vi "NI 5772 (AC) - Digitizer_(FPGA)Averaging (Working).vi"() -> ()   [LabVIEW 2020]
doc: "Example Description:\nThis example demonstrates how to enable Time Interleaved Sampling with the NI 5772 adapter module to achieve a sampling rate of 1.6GS/s. This example continuously acquires records of analog input data from the NI 5772 adapter module. It allows you to select an AI channel, trigger type, and record size. This VI must be compiled before it is run. \n\nRunning the VI:\nThis VI must be run from the NI 5772 - Getting Started (Host).vi. Refer to the host VI documentation for steps regarding running and configuring the FPGA VI. \n\nExecution Steps:\nRefer to the Block Diagram of this VI for execution comments."
uses:
  Controls/AI Trigger Type.ctl
  Controls/Aquire State.ctl
  <vilib>/Platform/TimedLoop/XDataNode/timing_clust.ctl
  <vilib>/Platform/TimedLoop/XDataNode/nitl_modes.ctl
  <vilib>/Platform/TimedLoop/XDataNode/wakeup.ctl
  Controls/DigitizerState.ctl
  <vilib>/rvi/Emulation/niFpgaGetClockAttributes.vi
  <vilib>/rvi/Emulation/niFpgaSctlEmulationGetInTimedLoop.vi
  <vilib>/rvi/Emulation/niFpgaEmulationReportErrorSimple.vi
  <vilib>/rvi/eio/common/nirviEmuTemplateMethod_errors.vi
  <vilib>/rvi/Emulation/niFpgaCriticalErrorInLSC.vi
  <vilib>/rvi/Emulation/niFpgaProcessEmulError.vi
  <vilib>/rvi/Emulation/niFpgaEmulationIsFPGAContextNoSignature.vi
  <vilib>/rvi/errors/niFpgaSetErrorForExecOnDevCompSimple.vi
  <vilib>/rvi/eio/common/nirviEmuReportErrorAndStop.vi
  <vilib>/rvi/DataTransferAndStorage/Container/Common/niFpgaContainerGetUniqueNameForEmu.vi
  <vilib>/rvi/FIFO/Fifo_Resource/nirvififoEmulationSetSize.vi
  <vilib>/rvi/FIFO/Fifo_Resource/nirviFifoEmulationQueueMgr.vi
  <instcachedir>/0/nirviFifoEmulationQueueMgr_E5CAEC123FF24DC58D834DCA3CDAA9B5.lvgen/nirviFifoEmulationQueueMgr_E5CAEC123FF24DC58D834DCA3CDAA9B5_000.vi
  <vilib>/Utility/error.llb/Clear Errors.vi
  <vilib>/rvi/FIFO/Fifo_Resource/nirvififoEmulationCreateLock.vi
  <vilib>/rvi/FIFO/Fifo_Resource/nirvififoEmulationObtainLock.vi
  <vilib>/rvi/FIFO/Fifo_Resource/nirvififoEmulationReleaseLock.vi
  <vilib>/rvi/occurrence/nirviWaitOnOccurrenceBase.vi
  <vilib>/rvi/errors/nirviReportUnexpectedCaseInternalError.vi
  <vilib>/rvi/errors/nirviReportUnexpectedCaseInternalError (U32).vi
  <instcachedir>/0/nirviFifoEmulationQueueMgr_E5CAEC123FF24DC58D834DCA3CDAA9B5.lvgen/nirviFifoEmulationQueueMgr_E5CAEC123FF24DC58D834DCA3CDAA9B5_003.vi
  <vilib>/rvi/FIFO/Fifo_Resource/nirvififoEmulationDetermineInputValidOut.vi
  <vilib>/rvi/Memory/Memory_Emulation/nirvimemoryFastEmulation.vi
  <vilib>/rvi/Memory/Memory_Emulation/nirvimemoryEmulation.vi
  <vilib>/rvi/interface/RandomDataEmulation/niFpgaRandomDataHandleErrors.vi
  <instcachedir>/0/nirviFifoEmulationQueueMgr_E5CAEC123FF24DC58D834DCA3CDAA9B5.lvgen/nirviFifoEmulationQueueMgr_E5CAEC123FF24DC58D834DCA3CDAA9B5_004.vi
  <instrlib>/_niInstr/Basic Elements/v1/FPGA/Private/Count Up U64.vi
  <vilib>/eio/EIONode/EIONode.xnode
  <vilib>/Platform/TimedLoop/XDataNode/XDataNode.xnode
  <vilib>/rvi/DataTransferAndStorage/Container/XNode/niFpgaContainer.xnode
  <vilib>/rvi/FIFO/Fifo_Resource/nirvififoEmulationRead.vi
  <vilib>/rvi/FIFO/Fifo_Resource/nirvififoEmulationWrite.vi
  <vilib>/rvi/interface/RandomDataEmulation/nirviRandomDataFpgaReadWriteTemplate.vi
  <vilib>/Platform/TimedLoop/XDataNode/XDNodeRunTimeDep.lvlib
  <instrlib>/_niInstr/Basic Elements/v1/FPGA/niInstr Basic Elements v1 FPGA.lvlib
panel:
  in  "Pulse Width Off [cycles]":u16=5
  in  "Pulse Width On [cycles]":u16=10
  out "Read Size (Host)":u16=512 caption="Samples Per Trigger" min=1 step=1
  out "Trig Count":u64
  in  "Clear Count":bool
  in  "TrigIn Simulate":bool
  in  "vi/nGenTrig":bool
  in  "Arm Trigger":bool
  out "F to H FIFO Overflow?":bool caption="FIFO Overflow?"
  out "DataAlignmentFIFO":bool
  out "Aq to Trans FIFO Overflow?":bool caption="FIFO Overflow?"
  in  "Requested Samples Per Pixel":u16=512 caption="Samples Per Trigger" min=1 step=1
  in  "AvgCount_powerOf2":i16=1
  in  "Delay (us)":sgl
  in  "WaveSampleCount":sgl=256.0 format="%#_13g"
  in  "Wave Sampling Rate":sgl=200000000.0 format="%#_6p"
  in  "Trigger Level":i16
  in  "Trigger Type":T1
  out "AvgCount":u16=1
  out "Delay after Trig [cycles]":u16
  out "1/8th Samples Per Trigger":u16=512 caption="Samples Per Trigger" min=1 step=1
  out "WaitForWave\nCompletion [cycles]":u16
  in  "User Command Commit":bool
  in  "User Command":u8
  out "User Command Idle":bool
  out "User Command Status":u8
  in  "User Data 0":u16
  in  "User Data 1":u8
  out "PLL Locked":bool
  out "User Error":bool
  out "Configured?":bool
  # "Trigger Settings"
  # "FIFO Status"
  # "Analog Input"
  # "Clock Configuration"
  # "Resource Configuration"
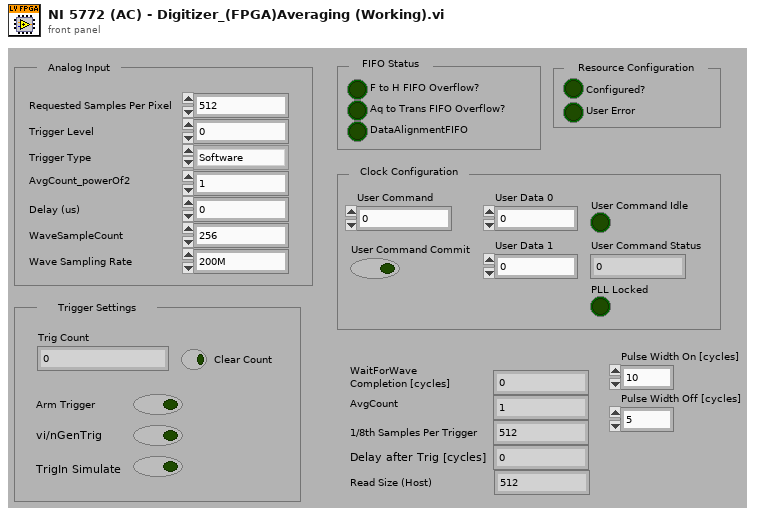
[diagram p1: front panel]
types:
  T1 = typedef "AI Trigger Type.ctl" = enum8{"Software", "Data Edge"}
  T2 = typedef "DigitizerState.ctl" = enum16{"Init", "Build/Clear Accumulator", "GetData", "SetData", "AverageCountCheck", "SendtoHost"}
  T3 = typedef "Aquire State.ctl" = enum8{"Idle", "Wait for Trigger", "AlignWave", "Hold Aquire", "Acquire", "WaitForWaveCompletion", "CheckAvg"}
  T4 = typedef "XDNodeRunTimeDep.lvlib/timing_clust.ctl" = cluster{"Expected End [f-1]":u64, "Actual End [f-1]":u64, "Finished Late? [f-1]":bool, "Expected End [i-1]":u64, "Actual End [i-1]":u64, "Finished Late? [i-1]":bool, "Expected Start [i]":u64, "Actual Start [i]":u64, "Expected Start [f]":u64, "Actual Start [f]":u64, "Source Name":string, "Structure Name":string, "Period":i64, "Deadline":i64, "Offset":i64, "Start":i64, "Priority":i32, "Timeout":i32, "Mode":T5, "Wakeup Reason":T6, "Error":errorcluster, "Source Type":string, "Secondary Source Type":string, "Global End Time":u64, "Global Start Time":u64, "Frame Duration":u64, "Iteration Duration":u64, "Assigned CPU":i32, "I/O Scan Engine Mode":u32}
  T5 = typedef "XDNodeRunTimeDep.lvlib/nitl_modes.ctl" = enum32{"No Change", "Process missed periods, maintain original phase", "Discard missed periods, maintain original phase", "Process missed periods, ignore original phase", "Discard missed periods, ignore original phase"}
  T6 = typedef "XDNodeRunTimeDep.lvlib/wakeup.ctl" = enum32{"Normal", "Aborted", "Asynchronous wakeup", "Timing source error", "Timed loop error", "Timeout"}
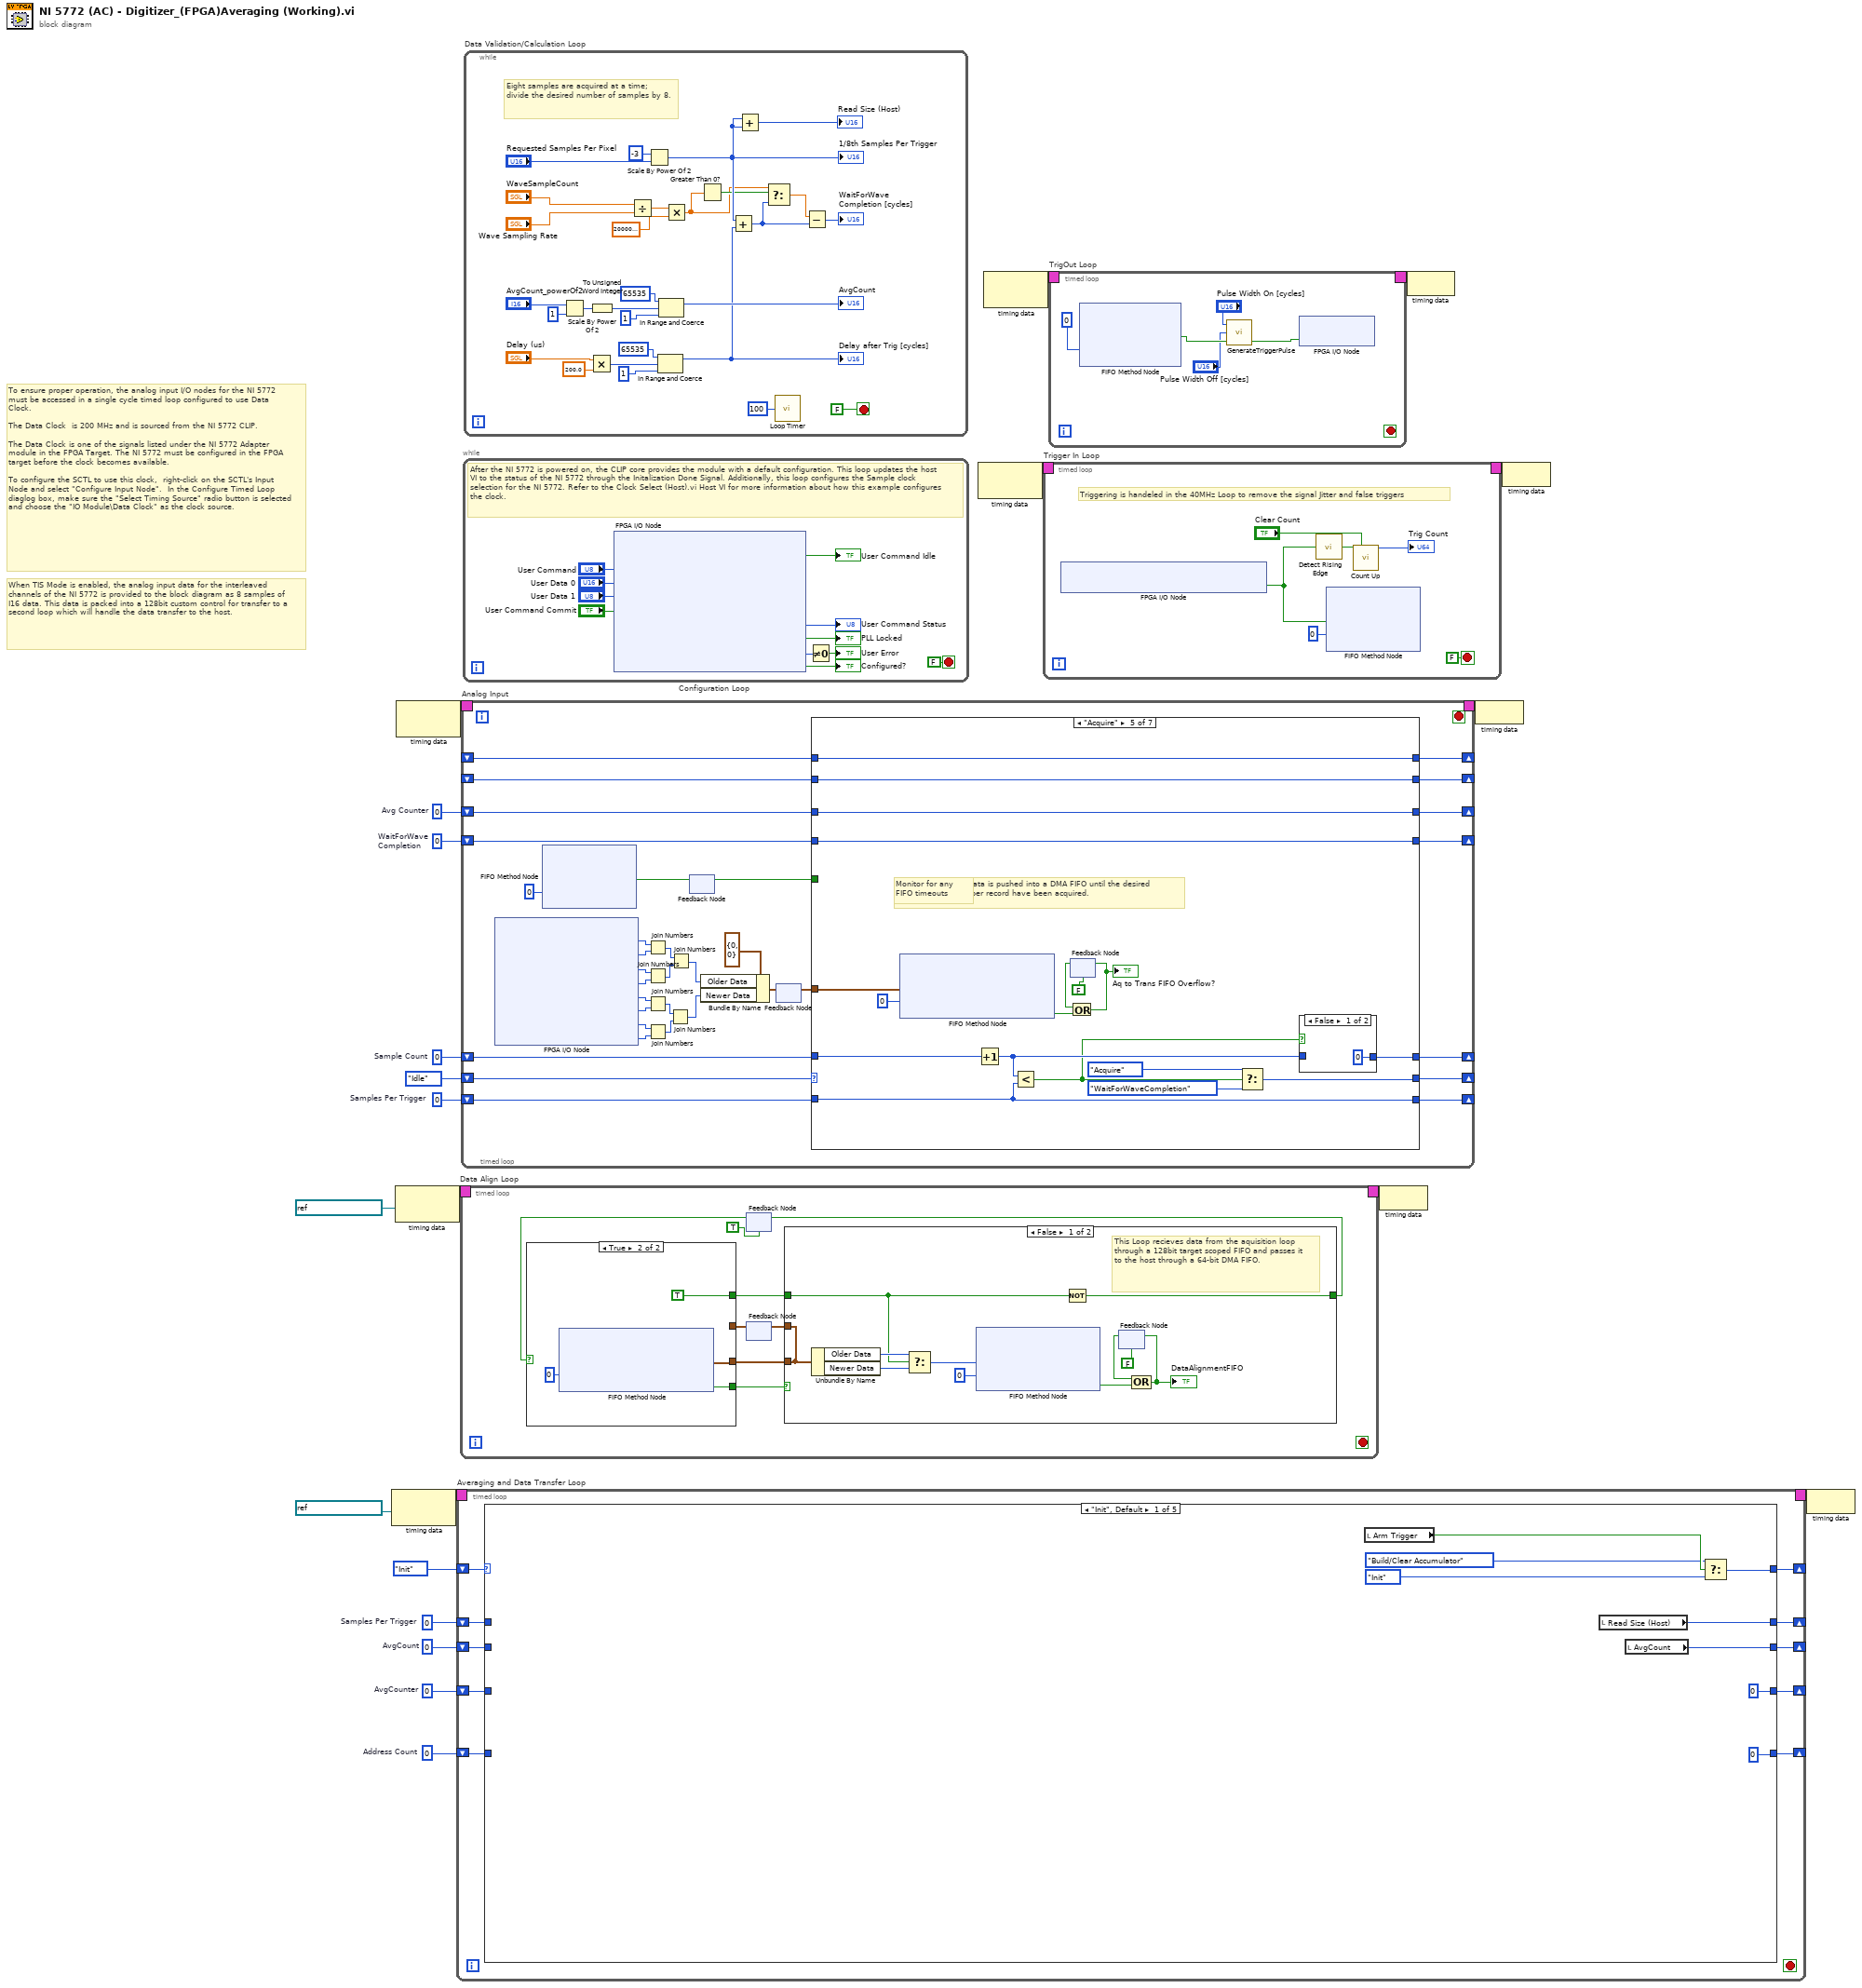
[diagram p0: block diagram]
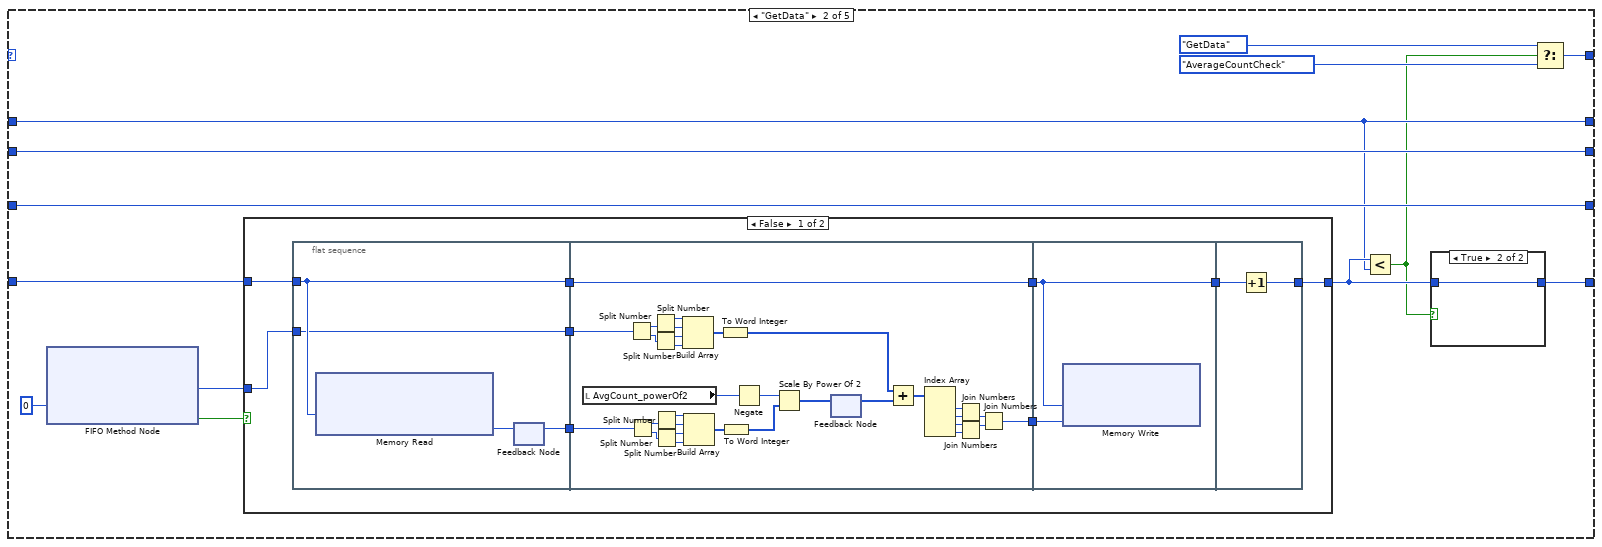
[diagram p2: hidden frame]
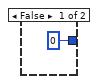
[diagram p3: hidden frame]
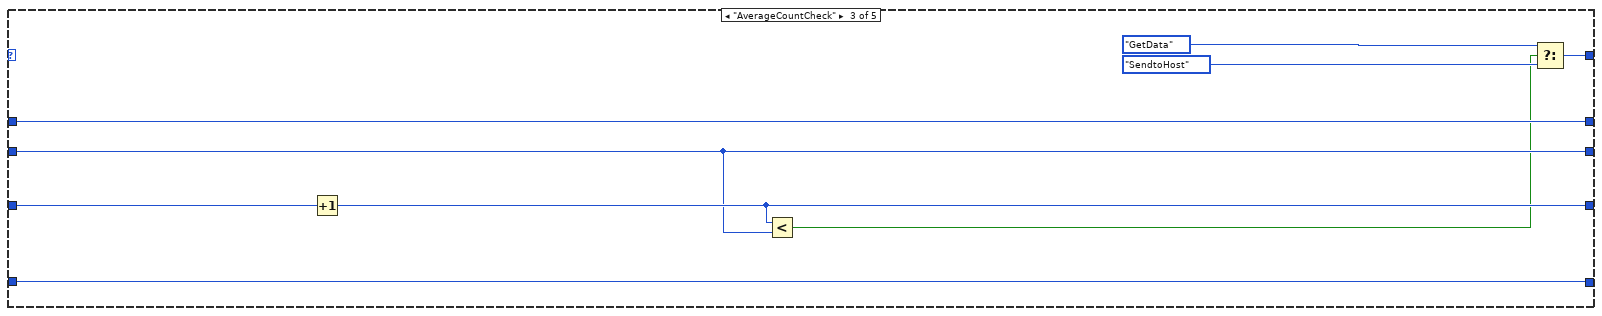
[diagram p5: hidden frame]
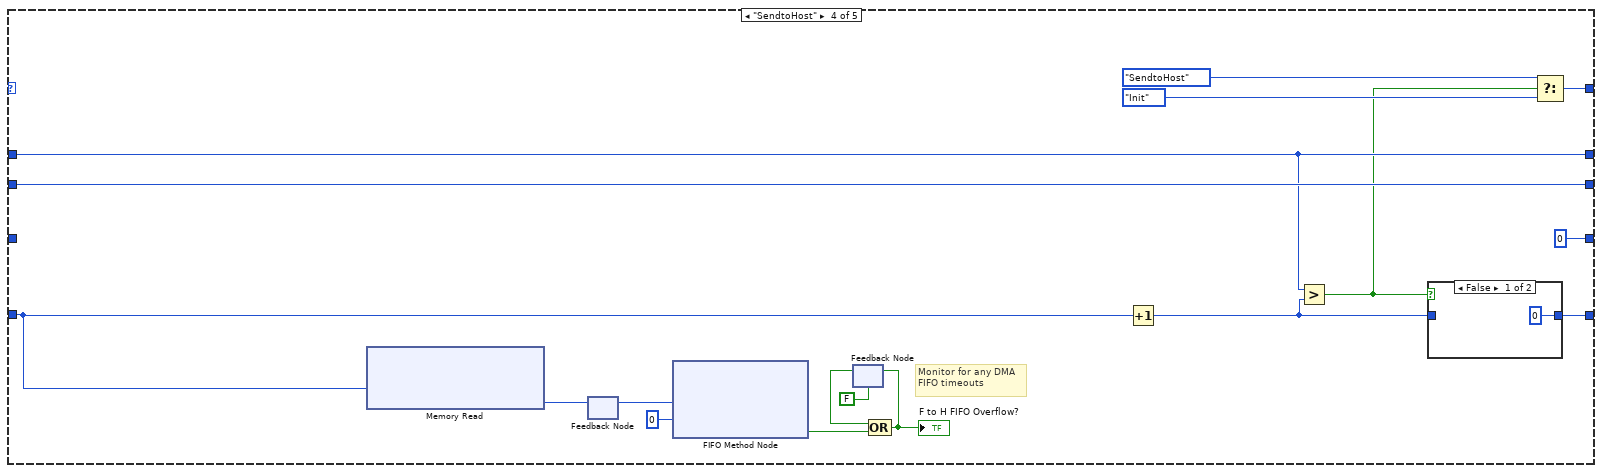
[diagram p6: hidden frame]
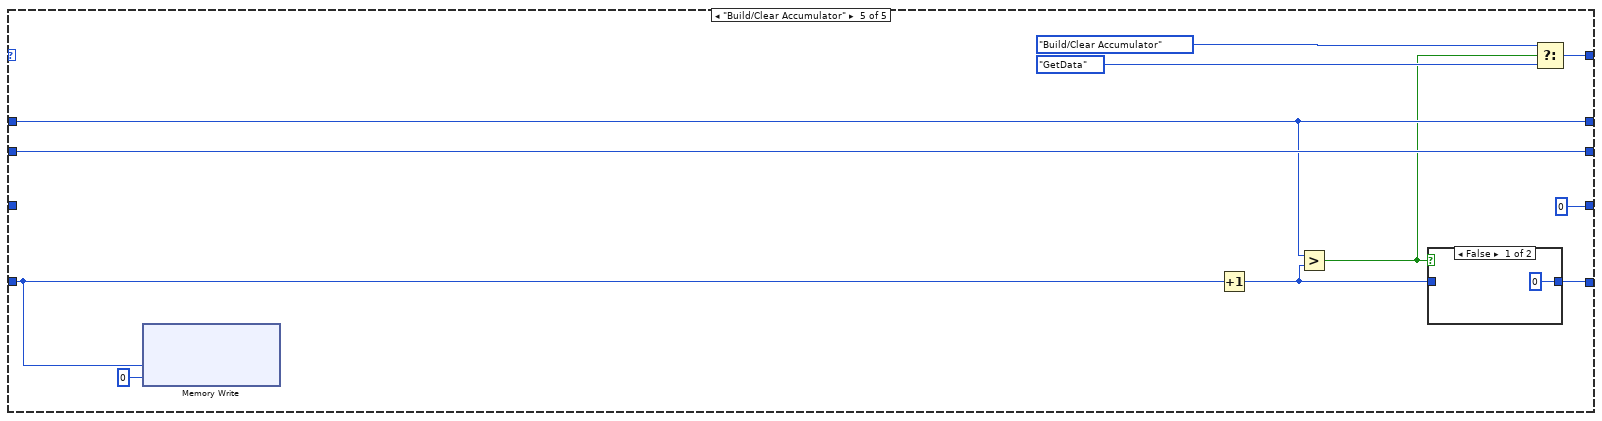
[diagram p8: hidden frame]
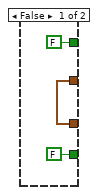
[diagram p10: hidden frame]
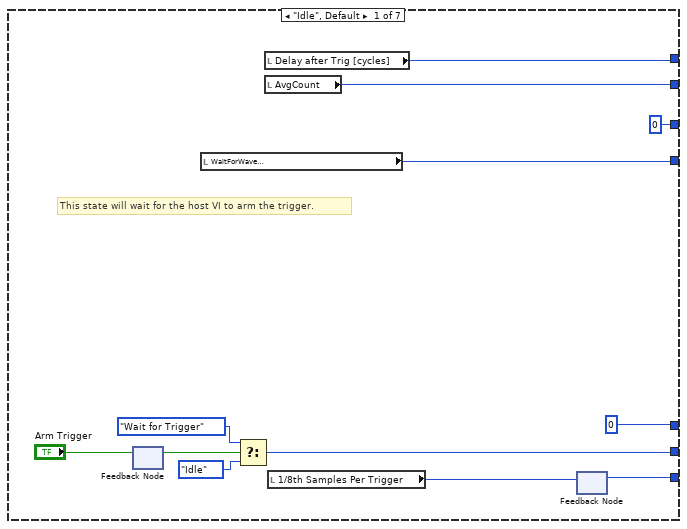
[diagram p12: hidden frame]
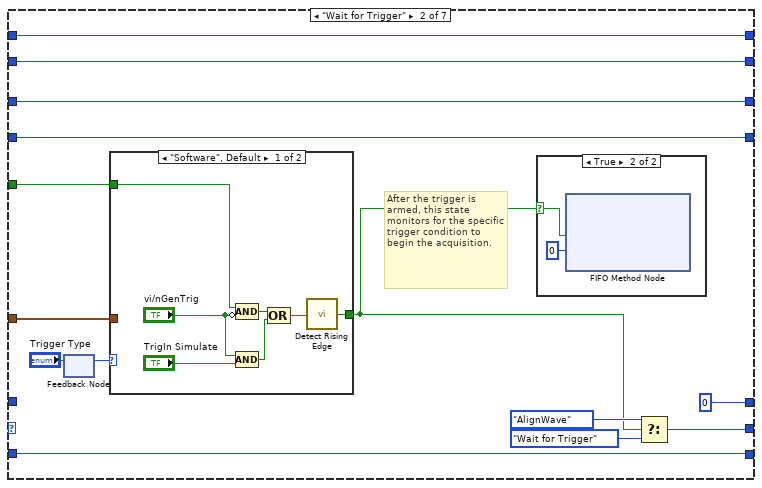
[diagram p13: hidden frame]
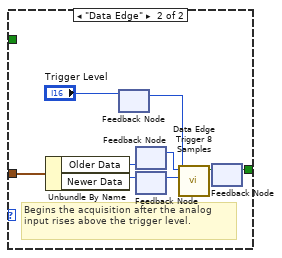
[diagram p15: hidden frame]
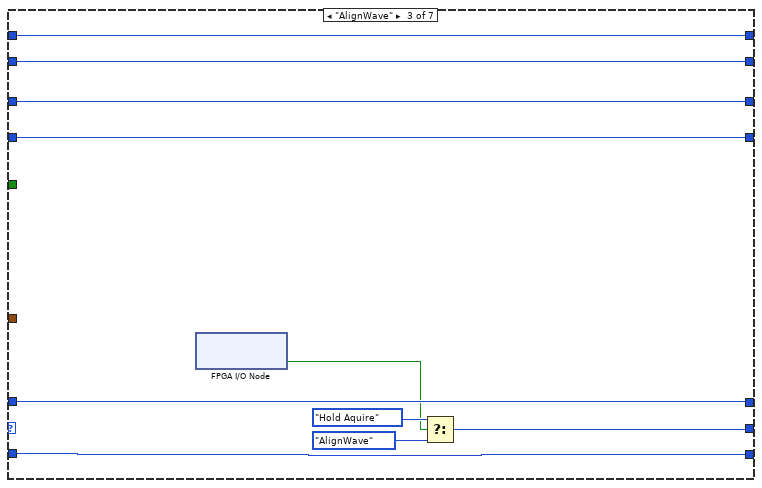
[diagram p16: hidden frame]
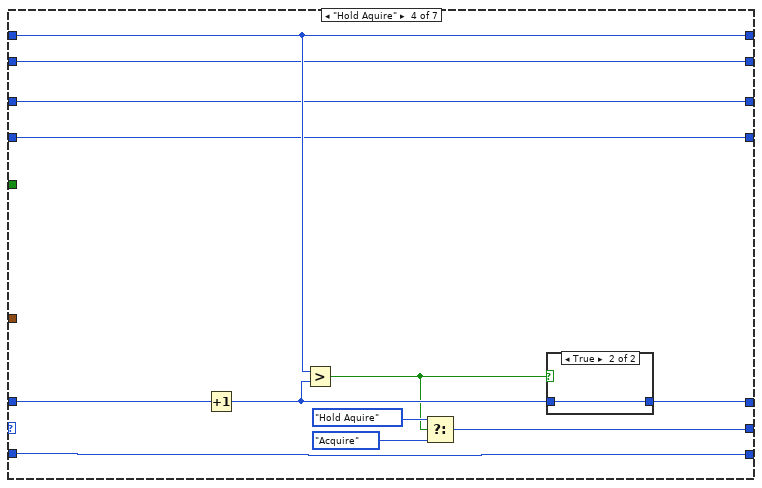
[diagram p17: hidden frame]
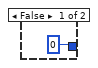
[diagram p18: hidden frame]
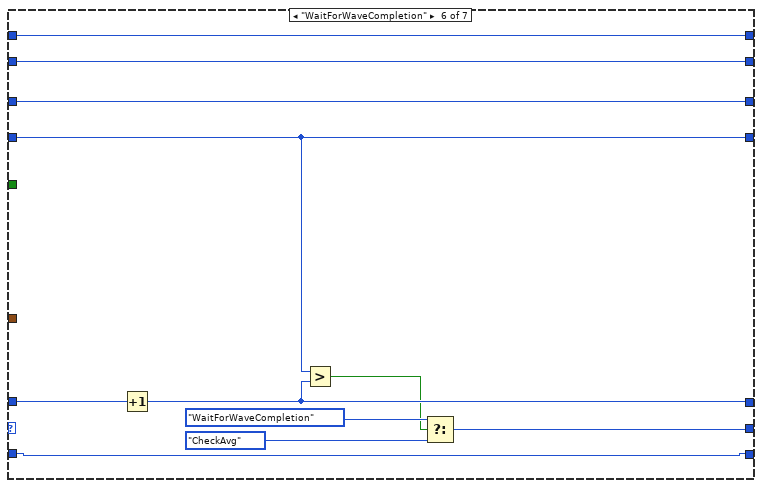
[diagram p20: hidden frame]
diagram:
  w8 = u16 0  # AvgCounter
  w7 = u32 0  # Address Count
  w6 = u16 0  # AvgCount
  w5 = u16 0  # Samples Per Trigger
  w14 = u16 0  # WaitForWave Completion
  w15 = u16 0  # Avg Counter
  w16 = u16 0  # Samples Per Trigger
  w17 = u16 0  # Sample Count
  # "When TIS Mode is enabled, the analog input data for the interleaved channels of the NI 5772 is provided to the block diagram as 8 samples of I16 data. This data is packed into a 128bit custom control for transfer to a second loop which will handle the data transfer to the host."
  # "To ensure proper operation, the analog input I/O nodes for the NI 5772 must be accessed in a single cycle timed loop configured to use Data Clock. \n\nThe Data Clock  is 200 MHz and is sourced from the NI 5772 CLIP.\n\nThe Data Clock is one of the signals listed under the NI 5772 Adapter module in the FPGA Target. The NI 5772 must be configured in the FPGA target before the clock becomes available. \n\nTo configure the SCTL to use this clock,  right-click on the SCTL's Input Node and select \"Configure Input Node\".  In the Configure Timed Loop diaglog box, make sure the \"Select Timing Source\" radio button is selected and choose the \"IO Module\\Data Clock\" as the clock source."
  n1 = node-c288(refnum<k21> "100 MHz Clock" ("Source Name")) -> (w10:T4)
  n2 = node-c288(refnum<k21> "100 MHz Clock" ("Source Name")) -> (w13:T4)
  n3 = node-c288() -> (w22:T4)  [unwired: 1 in]
  n4 = timed-loop "Averaging and Data Transfer Loop" {
    timing: w10 -> [_]
    timing-out: [_] -> w9
    shift-right: [w31] -> _
    shift-left: DigitizerState."Init" -> [w32]
    shift-right: [w30] -> _
    shift-left: w5 -> [w28]
    shift-right: [w29] -> _
    shift-left: w6 -> [w27]
    shift-right: [w25] -> _
    shift-left: w7 -> [w26]
    shift-right: [w23] -> _
    shift-left: w8 -> [w24]
    stop <- _ stop-if-true
    n5 = case shown="\"Init\", Default" w32 {
      tunnel: [w36 w51 w111 w127 w140] -> w31
      tunnel: [w34 w43 w109 w125 w138] -> w30
      tunnel: [w37 w50 w106 w130 w143] -> w29
      tunnel: w28 -> [_ w43 w109 w125 w138]
      tunnel: w27 -> [_ w50 w106 w130 w143]
      tunnel: w26 -> [_ w46 w110 w115 w134]
      tunnel: [u32 0 w45 w110 w126 w139] -> w25
      tunnel: [u16 0 w48 w107 u16 0 ("AvgCounter") u16 0 ("AvgCounter")] -> w23
      tunnel: w24 -> [_ w48 w108 _ _]
      frame "Init", Default {
        n6 = local read "Arm Trigger"() -> (w40:bool)
        n7 = local read "Read Size (Host)"() -> (w34:u16)
        n8 = local read "AvgCount"() -> (w37:u16)
        n9 = Select(t=DigitizerState."Build/Clear Accumulator", s=w40, f=DigitizerState."Init") -> (s? t:f=w36:T2)
      }
      frame "GetData" {
        n10 = xnode ("FIFO Method Node")("Timeout"=0) -> ("Element"=w47:u64, "Timed Out?"=w42:bool)  [unwired: 1 in, 1 out]
        n11 = case shown="False" w42 {
          tunnel: w47 -> [w61 _]
          tunnel: w46 -> [w63 w104]
          tunnel: [w60 w104] -> w44
          frame False {
            n12 = flat-sequence {
              tunnel: [w67] -> w64
              tunnel: w63 -> [w66]
              tunnel: w61 -> [w65]
              tunnel: [w66] -> w59
              tunnel: [w65] -> w57
              tunnel: w64 -> [w70]
              tunnel: [w89] -> w62
              tunnel: w59 -> [w88]
              tunnel: [w88] -> w58
              tunnel: w57 -> [w79]
              tunnel: w62 -> [w101]
              tunnel: w58 -> [w100]
              tunnel: [w100] -> w56
              tunnel: [w102] -> w60
              tunnel: w56 -> [w103]
              frame #0 {
                n13 = xnode ("Memory Read")("Address"=w66) -> ("Data"=w68:u64)  [unwired: 1 in, 1 out]
                n14 = feedback #1() -> (w67:u64)  [unwired: 1 in]
                n15 = feedback-in #1(w68) -> ()
              }
              frame #1 {
                n16 = local read "AvgCount_powerOf2"() -> (w98:i16)
                n17 = Split Number(x=w79) -> (hi(x)=w86:u32, lo(x)=w85:u32)
                n18 = Split Number(x=w70) -> (hi(x)=w71:u32, lo(x)=w72:u32)
                n19 = Split Number(x=w86) -> (hi(x)=w84:u16, lo(x)=w83:u16)
                n20 = Split Number(x=w85) -> (hi(x)=w82:u16, lo(x)=w81:u16)
                n21 = Split Number(x=w71) -> (hi(x)=w73:u16, lo(x)=w74:u16)
                n22 = Split Number(x=w72) -> (hi(x)=w75:u16, lo(x)=w76:u16)
                n23 = Build Array(w84, w83, w82, w81) -> (w80:u16[])
                n24 = Build Array(w73, w74, w75, w76) -> (w77:u16[])
                n25 = To Word Integer(number=w80) -> (16bit integer=w78:i16[])
                n26 = To Word Integer(number=w77) -> (16bit integer=w69:i16[])
                n27 = Negate(x=w98) -> (-x=w99:i16)
                n28 = Scale By Power Of 2(n=w99, x=w69) -> (x*2^n=w97:i16[])
                n29 = feedback-in #2(w97) -> ()
                n30 = feedback #2() -> (w87:i16[])  [unwired: 1 in]
                n31 = Add(x=w78, y=w87) -> (x+y=w90:i16[])
                n32 = Index Array(array=w90) -> (element #1=w93:i16, element #2=w94:i16, element #3=w95:i16, element #4=w96:i16)  [unwired: 4 in]
                n33 = Join Numbers(hi=w93, lo=w94) -> ((hi.lo)=w91:u32)
                n34 = Join Numbers(hi=w95, lo=w96) -> ((hi.lo)=w92:u32)
                n35 = Join Numbers(hi=w91, lo=w92) -> ((hi.lo)=w89:u64)
              }
              frame #2 {
                n36 = xnode ("Memory Write")("Address"=w100, "Data"=w101) -> ()  [unwired: 1 in, 1 out]
              }
              frame #3 {
                n37 = Increment(x=w103) -> (x+1=w102:u32)
              }
            }
          }
          frame True {
          }
        }
        n38 = Less?(x=w44, y=w43) -> (x < y?=w41:bool)
        n39 = case shown="True" w41 {
          tunnel: w44 -> [_ w55]
          tunnel: [u32 0 w55] -> w45
          frame False {
          }
          frame True {
          }
        }
        n40 = Select(t=DigitizerState."GetData", s=w41, f=DigitizerState."AverageCountCheck") -> (s? t:f=w51:T2)
      }
      frame "AverageCountCheck" {
        n41 = Increment(x=w108) -> (x+1=w107:u16)
        n42 = Less?(x=w107, y=w106) -> (x < y?=w105:bool)
        n43 = Select(t=DigitizerState."GetData", s=w105, f=DigitizerState."SendtoHost") -> (s? t:f=w111:T2)
      }
      frame "SendtoHost" {
        # "Monitor for any DMA FIFO timeouts"
        n44 = xnode ("Memory Read")("Address"=w115) -> ("Data"=w116:u64)  [unwired: 1 in, 1 out]
        n45 = feedback #3() -> (w114:u64)  [unwired: 1 in]
        n46 = feedback-in #3(w116) -> ()
        n47 = xnode ("FIFO Method Node")("Element"=w114, "Timeout"=0) -> ("Timed Out?"=w121:bool)  [unwired: 1 in, 1 out]
        n48 = feedback #4(FALSE) -> (w120:bool)
        n49 = Compound Arithmetic op=OR(w120, w121) -> (w122:bool)
        "F to H FIFO Overflow?" <- w122
        n50 = feedback-in #4(w122) -> ()
        n51 = Increment(x=w115) -> (x+1=w124:u32)
        n52 = Greater?(x=w125, y=w124) -> (0:w123:bool)
        n53 = case shown="False" w123 {
          tunnel: w124 -> [_ w132]
          tunnel: [u32 0 w132] -> w126
          frame False {
          }
          frame True {
          }
        }
        n54 = Select(t=DigitizerState."SendtoHost", s=w123, f=DigitizerState."Init") -> (s? t:f=w127:T2)
      }
      frame "Build/Clear Accumulator" {
        n55 = xnode ("Memory Write")("Address"=w134, "Data"=u64 0) -> ()  [unwired: 1 in, 1 out]
        n56 = Increment(x=w134) -> (x+1=w137:u32)
        n57 = Greater?(x=w138, y=w137) -> (0:w136:bool)
        n58 = case shown="False" w136 {
          tunnel: w137 -> [_ w145]
          tunnel: [u32 0 w145] -> w139
          frame False {
          }
          frame True {
          }
        }
        n59 = Select(t=DigitizerState."Build/Clear Accumulator", s=w136, f=DigitizerState."GetData") -> (s? t:f=w140:T2)
      }
    }
  }
  n60 = timed-loop "Data Align Loop" {
    timing: w13 -> [_]
    timing-out: [_] -> w12
    stop <- _ stop-if-true
    n61 = feedback #5(TRUE ("Timed Out?")) -> (w150:bool)
    n62 = feedback #6() -> (w151:cluster{"Older Data":u64, "Newer Data":u64})  [unwired: 1 in]
    n63 = case shown="True" w150 {
      tunnel: [w156 w159] -> w153
      tunnel: [FALSE ("Timed Out?") w160] -> w155
      tunnel: [FALSE ("Timed Out?") TRUE ("Timed Out?")] -> w154
      tunnel: w151 -> [w156 _]
      frame False {
      }
      frame True {
        n64 = xnode ("FIFO Method Node")("Timeout"=0) -> ("Element"=w159:cluster{"Older Data":u64, "Newer Data":u64}, "Timed Out?"=w160:bool)  [unwired: 1 in, 1 out]
      }
    }
    n65 = case shown="False" w155 {
      tunnel: [w171 w175] -> w149
      tunnel: w154 -> [w172 w175]
      tunnel: w153 -> [w170 w174]
      tunnel: [w170 w174] -> w152
      frame False {
        # "This Loop recieves data from the aquisition loop through a 128bit target scoped FIFO and passes it to the host through a 64-bit DMA FIFO."
        n66 = Unbundle By Name(w170) -> ("Older Data"=w173:u64, "Newer Data"=w169:u64)
        n67 = Select(t=w173, s=w172, f=w169) -> (s? t:f=w163:u64)
        n68 = xnode ("FIFO Method Node")("Element"=w163, "Timeout"=0) -> ("Timed Out?"=w165:bool)  [unwired: 1 in, 1 out]
        n69 = Not(x=w172) -> (.not. x?=w171:bool)
        n70 = feedback #7(FALSE) -> (w166:bool)
        n71 = Compound Arithmetic op=OR(w166, w165) -> (w164:bool)
        "DataAlignmentFIFO" <- w164
        n72 = feedback-in #7(w164) -> ()
      }
      frame True {
      }
    }
    n73 = feedback-in #5(w149) -> ()
    n74 = feedback-in #6(w152) -> ()
  }
  n75 = timed-loop "Analog Input" {
    timing: w22 -> [_]
    timing-out: [_] -> w21
    shift-right: [w210] -> _
    shift-left: Aquire_State."Idle" ("Acquire State") -> [w200]
    shift-right: [w211] -> _
    shift-left: w17 -> [w201]
    shift-right: [w209] -> _
    shift-left: w16 -> [w199]
    shift-right: [w186] -> _
    shift-left: _ -> [w185]
    shift-right: [w184] -> _
    shift-left: _ -> [w183]
    shift-right: [w181] -> _
    shift-left: w15 -> [w182]
    shift-right: [w179] -> _
    shift-left: w14 -> [w178]
    stop <- _ stop-if-true
    n76 = xnode "FPGA I/O Node"() -> ("IO Module\\AI 1 Data N-3"=w192:i16, "IO Module\\AI 0 Data N-3"=w191:i16, "IO Module\\AI 1 Data N-2"=w190:i16, "IO Module\\AI 0 Data N-2"=w189:i16, "IO Module\\AI 1 Data N-1"=w193:i16, "IO Module\\AI 0 Data N-1"=w194:i16, "IO Module\\AI 1 Data N"=w195:i16, "IO Module\\AI 0 Data N"=w196:i16)  [unwired: 8 in, 8 out]
    n77 = xnode ("FIFO Method Node")("Timeout"=0) -> ("Element"=w187:bool)  [unwired: 1 in, 2 out]
    n78 = Join Numbers(hi=w192, lo=w191) -> ((hi.lo)=w204:u32)
    n79 = Join Numbers(hi=w190, lo=w189) -> ((hi.lo)=w206:u32)
    n80 = Join Numbers(hi=w193, lo=w194) -> ((hi.lo)=w205:u32)
    n81 = Join Numbers(hi=w195, lo=w196) -> ((hi.lo)=w207:u32)
    n82 = Join Numbers(hi=w205, lo=w207) -> ((hi.lo)=w197:u64)
    n83 = Join Numbers(hi=w204, lo=w206) -> ((hi.lo)=w198:u64)
    n84 = feedback-in #8(w187) -> ()
    n85 = feedback #8() -> (w180:bool)  [unwired: 1 in]
    n86 = Bundle By Name(cluster=cluster{"Older Data":u64, "Newer Data":u64} {"Older Data"=0, "Newer Data"=0} ("Element"), "Older Data"=w198, "Newer Data"=w197) -> (w202:cluster{"Older Data":u64, "Newer Data":u64})
    n87 = feedback #9() -> (w208:cluster{"Older Data":u64, "Newer Data":u64})  [unwired: 1 in]
    n88 = feedback-in #9(w202) -> ()
    n89 = case shown="\"Acquire\"" w200 {
      tunnel: [u16 0 u16 0 w261 w273 w282 w304 u16 0] -> w211
      tunnel: w201 -> [_ _ w261 w272 w297 w306 _]
      tunnel: [w220 w232 w264 w276 w296 w309 w320] -> w210
      tunnel: [w217 w236 w262 w274 w293 w307 w318] -> w209
      tunnel: w199 -> [_ w236 w262 w274 w293 w307 w318]
      tunnel: w208 -> [_ w235 _ _ w292 _ _]
      tunnel: w180 -> [_ w230 _ _ _ _ _]
      tunnel: [w216 w228 w260 w271 w286 w305 w317] -> w186
      tunnel: w185 -> [_ w228 w260 w271 w286 w305 w317]
      tunnel: [w215 w227 w259 w269 w285 w302 w315] -> w184
      tunnel: w183 -> [_ w227 w259 w269 w285 w302 w315]
      tunnel: [u16 0 ("Avg Count") w226 w258 w268 w284 w301 w314] -> w181
      tunnel: w182 -> [_ w226 w258 w268 w284 w301 w316]
      tunnel: [w212 w224 w256 w266 w280 w300 w311] -> w179
      tunnel: w178 -> [_ w224 w256 w266 w280 w300 w311]
      frame "Idle", Default {
        # "This state will wait for the host VI to arm the trigger."
        n90 = feedback-in #10("Arm Trigger") -> ()
        n91 = feedback #10() -> (w218:bool)  [unwired: 1 in]
        n92 = local read "WaitForWave\nCompletion [cycles]"() -> (w212:u16)
        n93 = Select(t=Aquire_State."Wait for Trigger" ("Acquire State"), s=w218, f=Aquire_State."Idle" ("Acquire State")) -> (s? t:f=w220:T3)
        n94 = local read "Delay after Trig [cycles]"() -> (w216:u16)
        n95 = local read "AvgCount"() -> (w215:u16)
        n96 = local read "1/8th Samples Per Trigger"() -> (w213:u16)
        n97 = feedback-in #11(w213) -> ()
        n98 = feedback #11() -> (w217:u16)  [unwired: 1 in]
      }
      frame "Wait for Trigger" {
        # "After the trigger is armed, this state monitors for the specific trigger condition to begin the acquisition."
        n99 = feedback-in #12("Trigger Type") -> ()
        n100 = feedback #12() -> (w229:T1)  [unwired: 1 in]
        n101 = case shown="\"Software\", Default" w229 {
          tunnel: w235 -> [_ w255]
          tunnel: [w246 w247] -> w225
          tunnel: w230 -> [w241 _]
          frame "Software", Default {
            n102 = Compound Arithmetic op=AND(w241, invert "vi/nGenTrig") -> (w245:bool)
            n103 = Compound Arithmetic op=AND("vi/nGenTrig", "TrigIn Simulate") -> (w243:bool)
            n104 = Compound Arithmetic op=OR(w245, w243) -> (w240:bool)
            n105 = call <instrlib>:"Detect Rising Edge.vi"("signal"=w240) -> ("edge detected"=w246:bool)  [unwired: 14 in]
          }
          frame "Data Edge" {
            # "Begins the acquisition after the analog input rises above the trigger level."
            n106 = Unbundle By Name(w255) -> ("Older Data"=w253:u64, "Newer Data"=w251:u64)
            n107 = feedback-in #13("Trigger Level") -> ()
            n108 = feedback #13() -> (w249:i16)  [unwired: 1 in]
            n109 = feedback-in #14(w253) -> ()
            n110 = feedback #14() -> (w248:u64)  [unwired: 1 in]
            n111 = feedback-in #15(w251) -> ()
            n112 = feedback #15() -> (w250:u64)  [unwired: 1 in]
            n113 = call "Data Edge Trigger 8 Samples.vi"("Trigger Level"=w249, "Newer Data In"=w250, "Older Data In"=w248) -> ("Trigger"=w254:bool)  [unwired: 8 in]
            n114 = feedback-in #16(w254) -> ()
            n115 = feedback #16() -> (w247:bool)  [unwired: 1 in]
          }
        }
        n116 = case shown="True" w225 {
          selector: w225 -> [_ w239]
          frame False {
          }
          frame True {
            n117 = xnode ("FIFO Method Node")("Element"=w239, "Timeout"=0) -> ()  [unwired: 1 in, 2 out]
          }
        }
        n118 = Select(t=Aquire_State."AlignWave" ("Acquire State"), s=w225, f=Aquire_State."Wait for Trigger") -> (s? t:f=w232:T3)
      }
      frame "AlignWave" {
        n119 = xnode "FPGA I/O Node"() -> ("PXI_Trig0"=w257:bool)  [unwired: 1 in, 1 out]
        n120 = Select(t=Aquire_State."Hold Aquire" ("Acquire State"), s=w257, f=Aquire_State."AlignWave" ("Acquire State")) -> (s? t:f=w264:T3)
      }
      frame "Hold Aquire" {
        n121 = Increment(x=w272) -> (x+1=w270:u16)
        n122 = Greater?(x=w271, y=w270) -> (0:w267:bool)
        n123 = Select(t=Aquire_State."Hold Aquire" ("Acquire State"), s=w267, f=Aquire_State."Acquire" ("Acquire State")) -> (s? t:f=w276:T3)
        n124 = case shown="True" w267 {
          tunnel: [u16 0 w279] -> w273
          tunnel: w270 -> [_ w279]
          frame False {
          }
          frame True {
          }
        }
      }
      frame "Acquire" {
        # "Monitor for any  FIFO timeouts"
        # "While in this state, data is pushed into a DMA FIFO until the desired number of samples per record have been acquired."
        n125 = xnode ("FIFO Method Node")("Element"=w292, "Timeout"=0) -> ("Timed Out?"=w287:bool)  [unwired: 1 in, 1 out]
        n126 = Increment(x=w297) -> (x+1=w283:u16)
        n127 = Less?(x=w283, y=w293) -> (x < y?=w281:bool)
        n128 = feedback #17(FALSE) -> (w288:bool)
        n129 = Or(x=w288, y=w287) -> (x .or. y?=w289:bool)
        "Aq to Trans FIFO Overflow?" <- w289
        n130 = feedback-in #17(w289) -> ()
        n131 = Select(t=Aquire_State."Acquire" ("Acquire State"), s=w281, f=Aquire_State."WaitForWaveCompletion" ("Acquire State")) -> (s? t:f=w296:T3)
        n132 = case shown="False" w281 {
          tunnel: w283 -> [_ w299]
          tunnel: [u16 0 w299] -> w282
          frame False {
          }
          frame True {
          }
        }
      }
      frame "WaitForWaveCompletion" {
        n133 = Increment(x=w306) -> (x+1=w304:u16)
        n134 = Greater?(x=w300, y=w304) -> (0:w303:bool)
        n135 = Select(t=Aquire_State."WaitForWaveCompletion" ("Acquire State"), s=w303, f=Aquire_State."CheckAvg" ("Acquire State")) -> (s? t:f=w309:T3)
      }
      frame "CheckAvg" {
        n136 = Increment(x=w316) -> (x+1=w314:u16)
        n137 = Greater?(x=w315, y=w314) -> (0:w312:bool)
        n138 = Select(t=Aquire_State."AlignWave" ("Acquire State"), s=w312, f=Aquire_State."Idle") -> (s? t:f=w320:T3)
        n139 = xnode ("FIFO Method Node")("Element"=w312, "Timeout"=0) -> ()  [unwired: 1 in, 2 out]
      }
    }
  }
  n140 = while "Configuration Loop" {
    stop <- FALSE stop-if-true
    # "After the NI 5772 is powered on, the CLIP core provides the module with a default configuration. This loop updates the host VI to the status of the NI 5772 through the Initalization Done Signal. Additionally, this loop configures the Sample clock selection for the NI 5772. Refer to the Clock Select (Host).vi Host VI for more information about how this example configures the clock."
    n141 = xnode "FPGA I/O Node"("IO Module\\User Command"="User Command", "IO Module\\User Data 0"="User Data 0", "IO Module\\User Data 1"="User Data 1", "IO Module\\User Command Commit"="User Command Commit") -> ("IO Module\\User Command Idle"=→"User Command Idle":bool, "IO Module\\User Command Status"=→"User Command Status":u8, "IO Module\\PLL Locked"=→"PLL Locked":bool, "IO Module\\User Error"=w330:u8, "IO Module\\Initialization Done"=→"Configured?":bool)  [unwired: 9 in, 9 out]
    n142 = Not Equal To 0?(x=w330) -> (x != 0?=→"User Error":bool)
  }
  n143 = while "Data Validation/Calculation Loop" {
    stop <- FALSE stop-if-true
    # "Eight samples are acquired at a time; divide the desired number of samples by 8."
    n144 = Scale By Power Of 2(n="AvgCount_powerOf2", x=1 ("Timeout")) -> (x*2^n=w361:i32)
    n145 = To Unsigned Word Integer(number=w361) -> (unsigned 16bit integer=w358:u16)
    n146 = Multiply(x="Delay (us)", y=sgl 200.0) -> (x*y=w354:u16)
    n147 = Divide(x="WaveSampleCount", y="Wave Sampling Rate") -> (x/y=w346:sgl)
    n148 = Scale By Power Of 2(n=i16 -3, x="Requested Samples Per Pixel") -> (x*2^n=w340:u16)
    "1/8th Samples Per Trigger" <- w340
    n149 = In Range and Coerce(upper limit=u16 65535, x=w354, lower limit=u16 1) -> (coerced(x)=w347:u16)  [unwired: 1 out]
    "Delay after Trig [cycles]" <- w347
    n150 = In Range and Coerce(upper limit=u16 65535, x=w358, lower limit=u16 1) -> (coerced(x)=→"AvgCount":u16)  [unwired: 1 out]
    n151 = Multiply(x=w346, y=sgl 200000000.0) -> (x*y=w337:sgl)
    n152 = Greater Than 0?(x=w337) -> (x > 0?=w338:bool)
    n153 = Add(x=w340, y=w347) -> (x+y=w336:u16)
    n154 = Add(x=w340, y=w340) -> (x+y=→"Read Size (Host)":u16)
    n155 = Select(t=w337, s=w338, f=w336) -> (s? t:f=w339:sgl)
    n156 = call "Loop Timer"("Count(uSec)"=u32 100 ("Count(mSec)")) -> ()  [unwired: 1 out]
    n157 = Subtract(x=w339, y=w336) -> (x-y=→"WaitForWave\nCompletion [cycles]":u16)
  }
  n158 = node-c288() -> (w20:T4)  [unwired: 1 in]
  n159 = node-c288() -> (w2:T4)  [unwired: 1 in]
  n160 = timed-loop "Trigger In Loop" {
    timing: w20 -> [_]
    timing-out: [_] -> w19
    stop <- FALSE stop-if-true
    # "Triggering is handeled in the 40MHz Loop to remove the signal Jitter and false triggers"
    n161 = xnode "FPGA I/O Node"() -> ("IO Module\\Asynchronous Trigger Input"=w369:bool)  [unwired: 1 in, 1 out]
    n162 = call <instrlib>:"Detect Rising Edge.vi"("signal"=w369) -> ("edge detected"=w366:bool)  [unwired: 14 in]
    n163 = xnode ("FIFO Method Node")("Element"=w369, "Timeout"=0) -> ()  [unwired: 1 in, 2 out]
    n164 = call-poly <instrlib>:"Count Up.vi"("increment"=w366, "reset"="Clear Count") -> ("count out"=→"Trig Count":u64)  [unwired: 13 in]
  }
  n165 = timed-loop "TrigOut Loop" {
    timing: w2 -> [_]
    timing-out: [_] -> w1
    stop <- _ stop-if-true
    n166 = xnode ("FIFO Method Node")("Timeout"=0) -> ("Element"=w375:bool)  [unwired: 1 in, 2 out]
    n167 = call "GenerateTriggerPulse.vi"("Trigger"=w375, "Pulse Width Off [cycles]"="Pulse Width Off [cycles]", "Pulse Width On [cycles]"="Pulse Width On [cycles]") -> ("Out"=w374:bool)  [unwired: 2 out]
    n168 = xnode "FPGA I/O Node"("PXI_Trig1"=w374) -> ()  [unwired: 1 in, 1 out]
  }
  n169 = node-c288(w12) -> ()
  n170 = node-c288(w1) -> ()
  n171 = node-c288(w21) -> ()
  n172 = node-c288(w19) -> ()
  n173 = node-c288(w9) -> ()
